vi "Day 14-1.vi"() -> ()   [LabVIEW 2020]
panel:
  out "Numeric":i32
  out "x-y":u64
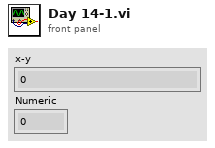
[diagram p1: front panel]
types:
  T1 = typedef "Puzzle 14.ctl" = cluster{"Sequence":u8[], "Histogram":u64[], "Map":map{u8[], u8}}
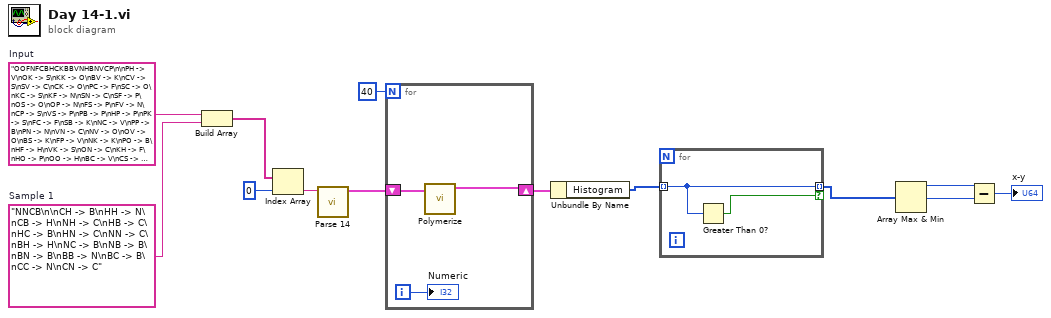
[diagram p0: block diagram]
diagram:
  w12 = "NNCB\n\nCH -> B\nHH -> N\nCB -> H\nNH -> C\nHB -> C\nHC -> B\nHN -> C\nNN -> C\nBH -> H\nNC -> B\nNB -> B\nBN -> B\nBB -> N\nBC -> B\nCC -> N\nCN -> C"  # Sample 1
  w13 = "OOFNFCBHCKBBVNHBNVCP\n\nPH -> V\nOK -> S\nKK -> O\nBV -> K\nCV -> S\nSV -> C\nCK -> O\nPC -> F\nSC -> O\nKC -> S\nKF -> N\nSN -> C\nSF -> P\nOS -> O\nOP -> N\nFS -> P\nFV -> N\nCP -> S\nVS -> P\nPB -> P\nHP -> P\nPK -> S\nFC -> F\nSB -> K\nNC -> V\nPP -> B\nPN -> N\nVN -> C\nNV -> O\nOV -> O\nBS -> K\nFP -> V\nNK -> K\nPO -> B\nHF -> H\nVK -> S\nON -> C\nKH -> F\nHO -> P\nOO -> H\nBC -> V\nCS -> O\nOC -> B\nVB -> N\nOF -> P\nFK -> H\nOH -> H\nCF -> K\nCC -> V\nBK -> O\nBH -> F\nVV -> N\nKS -> V\nFO -> F\nSH -> F\nOB -> O\nVH -> F\nHH -> P\nPF -> C\nNF -> V\nVP -> S\nCN -> V\nSK -> O\nFB -> S\nFN -> S\nBF -> H\nFF -> V\nCB -> P\nNN -> O\nVC -> F\nHK -> F\nBO -> H\nKO -> C\nCH -> N\nKP -> C\nHS -> P\nNP -> O\nNS -> V\nNB -> H\nHN -> O\nBP -> C\nVF -> S\nKN -> P\nHC -> C\nPS -> K\nBB -> O\nNO -> N\nNH -> F\nBN -> F\nKV -> V\nSS -> K\nCO -> H\nKB -> P\nFH -> C\nSP -> C\nSO -> V\nPV -> S\nVO -> O\nHV -> N\nHB -> V"  # Input
  n1 = Build Array(w13, w12) -> (w11:string[])
  n2 = Index Array(array=w11, index=0) -> (element=w9:string)
  n3 = call "Parse 14.vi"("String"=w9) -> ("Puzzle"=w8:T1)  [unwired: 10 in]
  n4 = for {
    N: 40 -> [_]
    shift-right: [w15] -> w6
    shift-left: w8 -> [w16]
    i -> [w14]
    n5 = call "Polymerize.vi"("Puzzle In"=w16) -> ("Puzzle"=w15:T1)  [unwired: 10 in]
    "Numeric" <- w14
  }
  n6 = Unbundle By Name(w6) -> ("Histogram"=w2:u64[])
  n7 = for {
    tunnel: w2 -> [w18] mode=indexing
    tunnel: [w18] -> w1 mode=indexing if=w17
    n8 = Greater Than 0?(x=w18) -> (x > 0?=w17:bool)
  }
  n9 = Array Max & Min(array=w1) -> (max value=w5:u64, min value=w4:u64)  [unwired: 2 out]
  n10 = Subtract(x=w5, y=w4) -> (x-y=→"x-y":u64)
